vi "断电保存变量.vi"() -> ()   [LabVIEW 2016, in "斯坦道多参数.lvlib"]
panel:
  in  "水样测试组数":dbl=1.0 caption="水样测试组数:"
  in  "水样稳定时间":dbl=5.0 caption="水样稳定时间:"
  in  "滤波设置":T1={"pH"=2, "DO"=2, "Cond"=2, "Turb"=2, "叶绿素a"=2, "藻密度"=2, "ORP"=2}
  in  "ORP参数":T2
  in  "藻密度参数":T2
  in  "叶绿素参数":T2
  in  "浊度参数":T2
  in  "电导率参数":T2
  in  "溶解氧参数":T2
  in  "PH参数":T2
  in  "水温参数":T2
  in  "orp":bool
  in  "orp标液1":dbl
  in  "电导率标液2":dbl
  in  "电导率标液1":dbl
  in  "pH标液2":dbl
  in  "pH标液1":dbl
  in  "自动断线重连":bool=TRUE
  in  "藻密度":bool
  in  "连接方式":u16(ring)=1 items=["Modbus RTU", "Modbus TCP"]
  in  "IP":string="192.168.1.206" caption="IP:"
  in  "Port":u16=502 caption="Port:"
  in  "定时控制输入":T3
  in  "探头选择":T4={"pH探头选择"=1, "DO探头选择"=1, "电导率探头选择"=1, "浊度探头选择"=1, "叶绿素a探头选择"=2, "蓝绿藻探头选择"=2, "orp探头选择"=1} {"orp探头选择" items=["禹山", "国弘", "纳清"]; "蓝绿藻探头选择" items=["禹山", "国弘", "纳清"]; "叶绿素a探头选择" items=["禹山", "国弘", "纳清"]; "浊度探头选择" items=["禹山", "国弘", "纳清"]; "电导率探头选择" items=["禹山", "国弘", "纳清"]; "DO探头选择" items=["禹山", "国弘", "纳清"]; "pH探头选择" items=["禹山", "国弘", "纳清"]}
  in  "蓝绿藻":bool
  in  "盐度自动获取":bool=TRUE
  out "大气压补偿":dbl=101.35
  out "盐度补偿":dbl
  in  "浊度标液2":dbl
  in  "浊度标液1":dbl
  in  "DO标液2":dbl=100.0
  in  "DO标液1":dbl
  in  "叶绿素a标液2":dbl
  in  "叶绿素a标液1":dbl
  in  "pH温度偏移补偿":dbl
  in  "Turb温度偏移补偿":dbl
  in  "Cond温度偏移补偿":dbl
  in  "DO温度偏移补偿":dbl
  in  "叶绿素a启用":bool
  in  "标样核查配置":T5={"数据保存间隔"=1.0, "保存组数"=5.0, "水温标样值"=0.0, "pH标样值"=0.0, "溶解氧标样值"=0.0, "电导率标样值"=0.0, "浊度标样值"=0.0, "pH启用"=FALSE, "溶解氧启用"=FALSE, "电导率启用"=FALSE, "浊度启用"=FALSE}
  in  "Temp":bool=TRUE
  in  "Cond":bool=TRUE
  in  "Turb":bool=TRUE
  in  "DO":bool=TRUE
  in  "pH":bool=TRUE
  in  "VISA资源名称":refnum<visa-resource-name>
  in  "水温通道":enum16{"pH", "Cond", "DO", "Turb"}(ring)
  # "请设置串口参数"
  # "请选择要启用的参数"
  # "组"
  # "min"
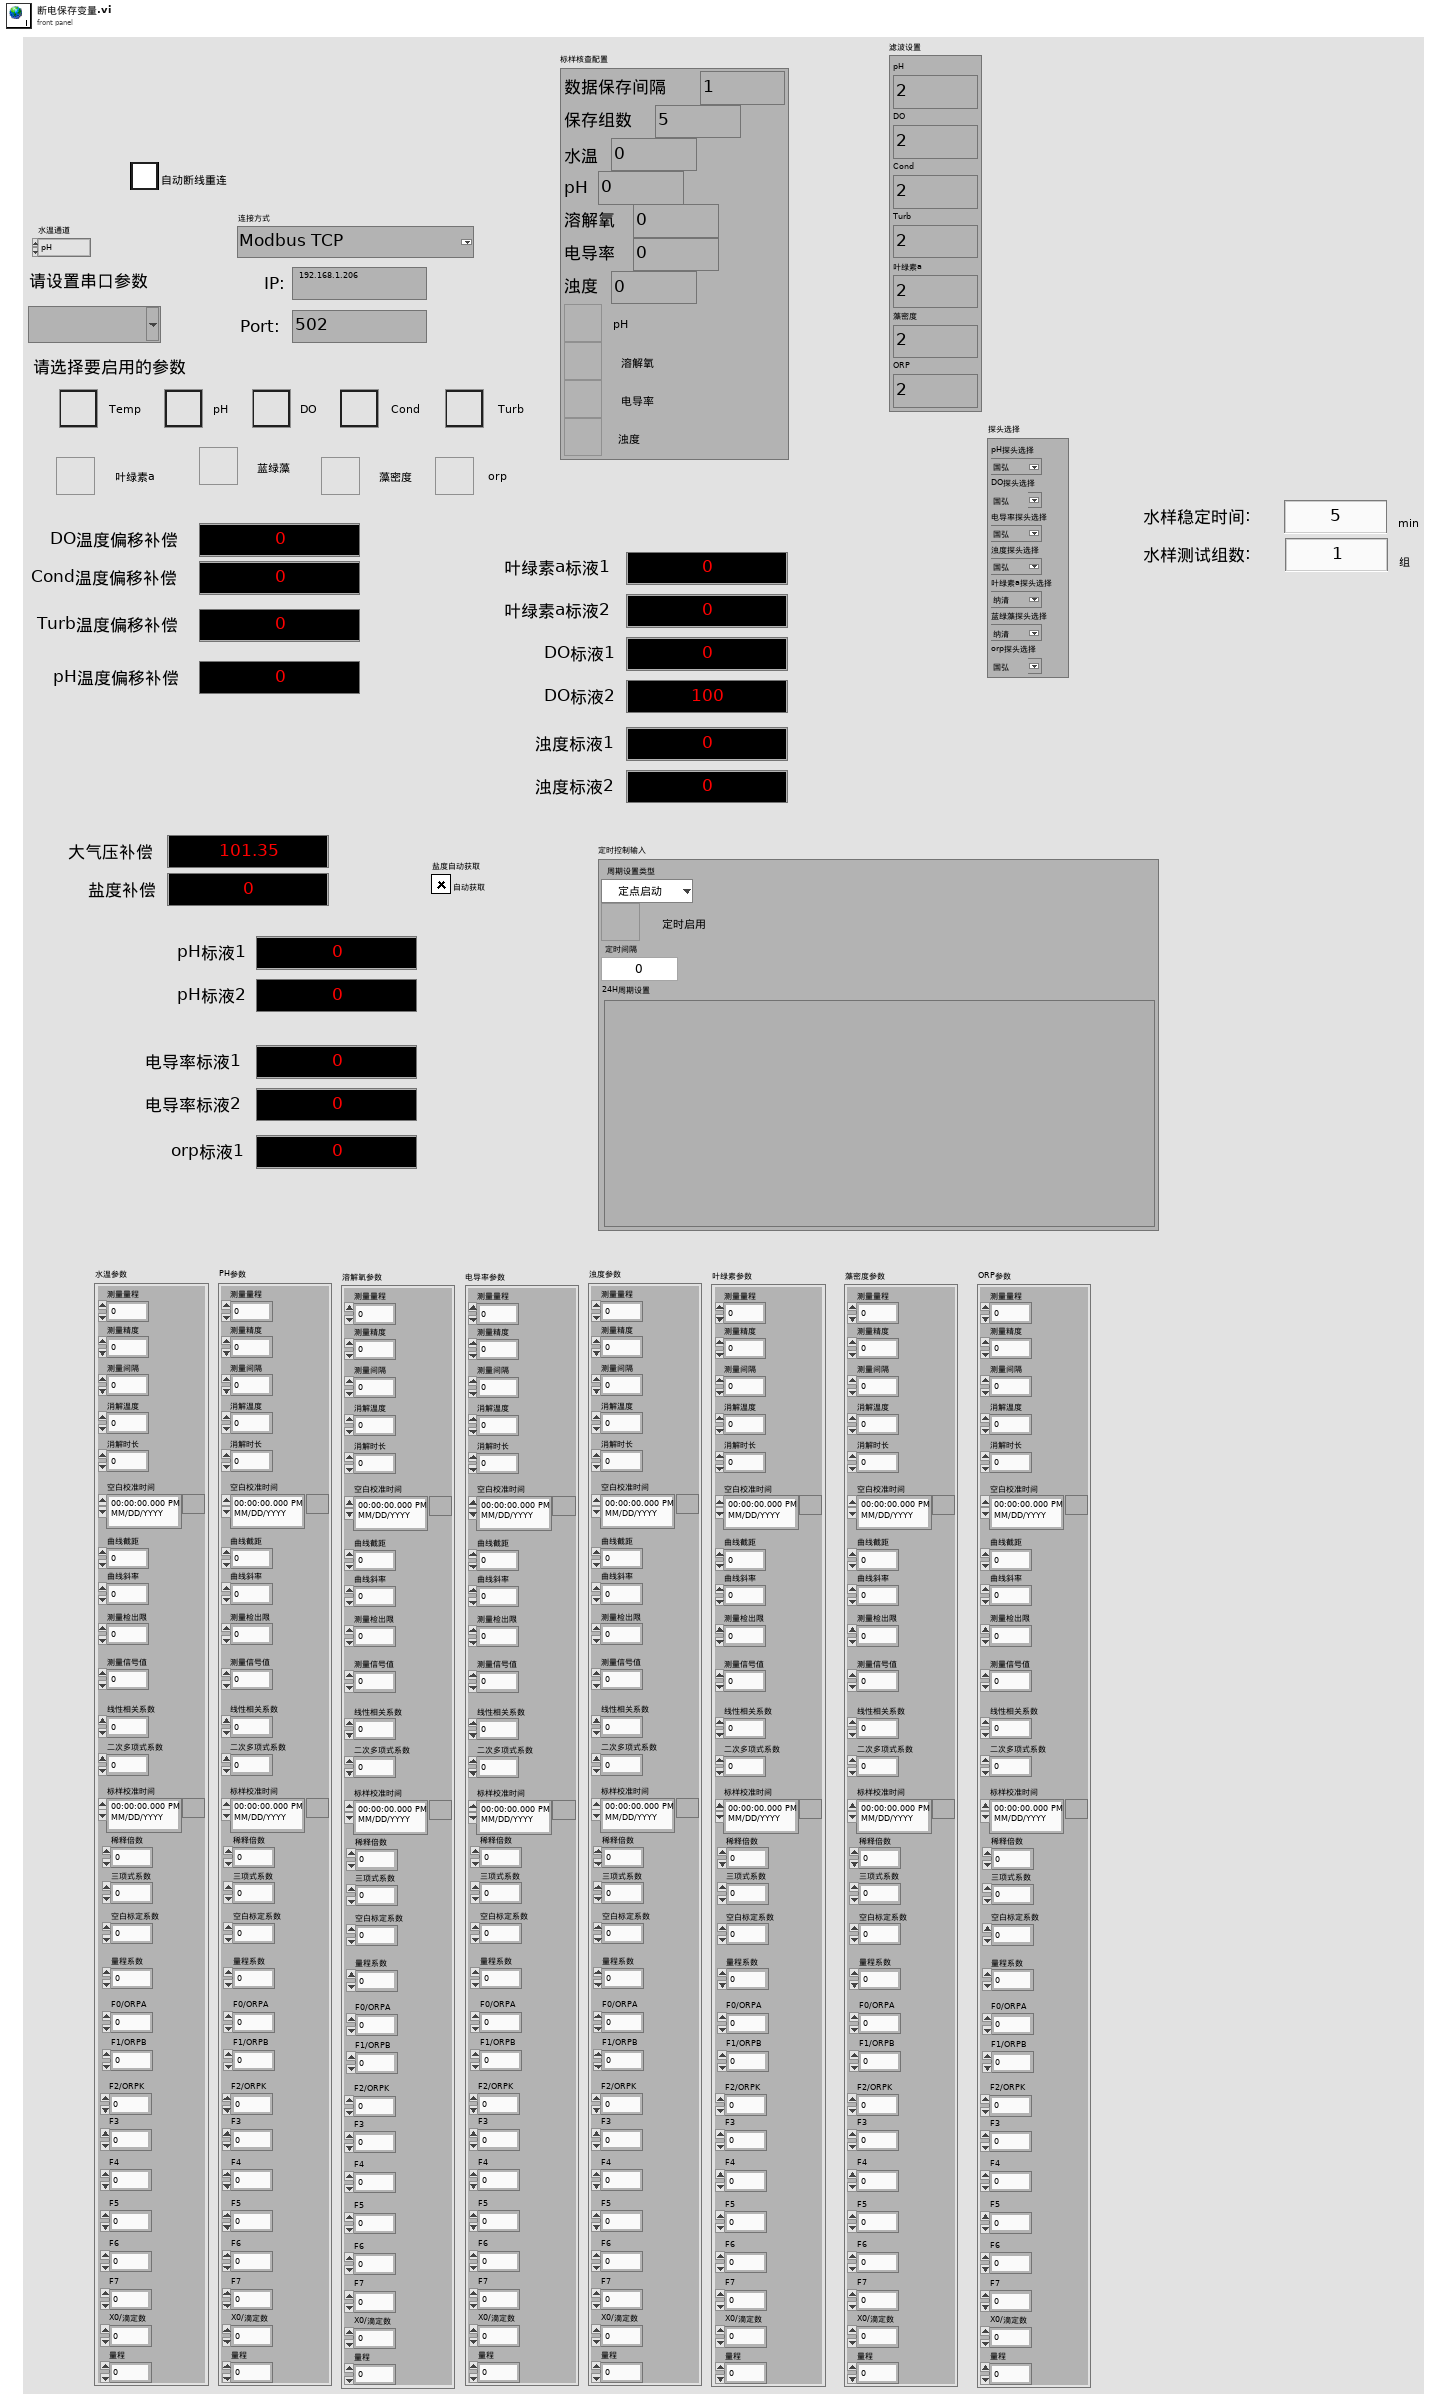
[diagram p1: front panel]
types:
  T1 = cluster{"pH":u32, "DO":u32, "Cond":u32, "Turb":u32, "叶绿素a":u32, "藻密度":u32, "ORP":u32}
  T2 = cluster{"测量量程":dbl, "测量精度":dbl, "测量间隔":dbl, "消解温度":dbl, "消解时长":dbl, "空白校准时间":timestamp, "曲线截距":dbl, "曲线斜率":dbl, "测量检出限":dbl, "测量信号值":dbl, "线性相关系数":dbl, "二次多项式系数":dbl, "标样校准时间":timestamp, "稀释倍数":dbl, "三项式系数":dbl, "空白标定系数":dbl, "量程系数":dbl, "F0/ORPA":dbl, "F1/ORPB":dbl, "F2/ORPK":dbl, "F3":dbl, "F4":dbl, "F5":dbl, "F6":dbl, "F7":dbl, "X0/滴定数":dbl, "量程":dbl}
  T3 = cluster{"周期设置类型":enum16{"定点启动", "间隔启动"}, "定时功能启用":bool, "定时间隔":u32, "24H周期设置":bool[]}
  T4 = cluster{"pH探头选择":u16, "DO探头选择":u16, "电导率探头选择":u16, "浊度探头选择":u16, "叶绿素a探头选择":u16, "蓝绿藻探头选择":u16, "orp探头选择":u16}
  T5 = cluster{"数据保存间隔":dbl, "保存组数":dbl, "水温标样值":dbl, "pH标样值":dbl, "溶解氧标样值":dbl, "电导率标样值":dbl, "浊度标样值":dbl, "pH启用":bool, "溶解氧启用":bool, "电导率启用":bool, "浊度启用":bool}
diagram:
